vi "testExample_ADC.vi"(8 "error in (no error)":errorcluster, 11 "TestCase in":refnum<class "MyTestCase_shido.lvclass">) -> (0 "error out":errorcluster, 3 "TestCase out":refnum<class "MyTestCase_shido.lvclass">)   [LabVIEW 2020, in "MyTestCase_shido.lvclass"]
doc: "Testea el ejemplo de leer adc de un dispositivo simulado en donde la respuesta esta previamente configurada."
uses:
  MyTestCase_shido.lvclass
  Implementacion/Simulated/Simulated.lvclass
  <vilib>/addons/_JKI Toolkits/VI Tester/TestCase.llb/TestCase.lvclass
  C:/Program Files/National Instruments/LabVIEW 2020/vi.lib/addons/_JKI Toolkits/VI Tester/TestCase.llb/TestCase.lvclass
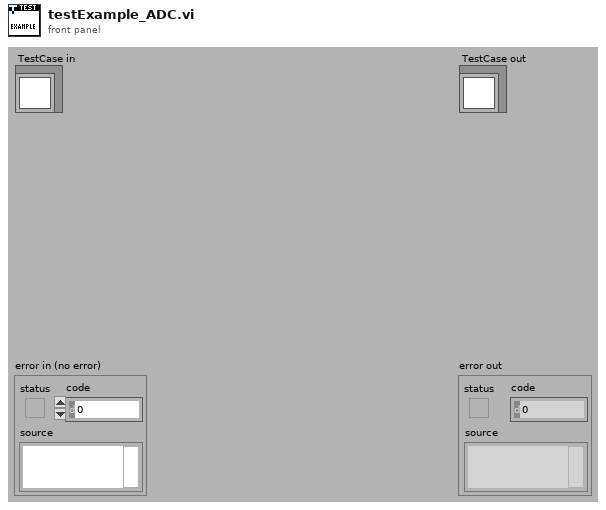
[diagram p1: front panel]
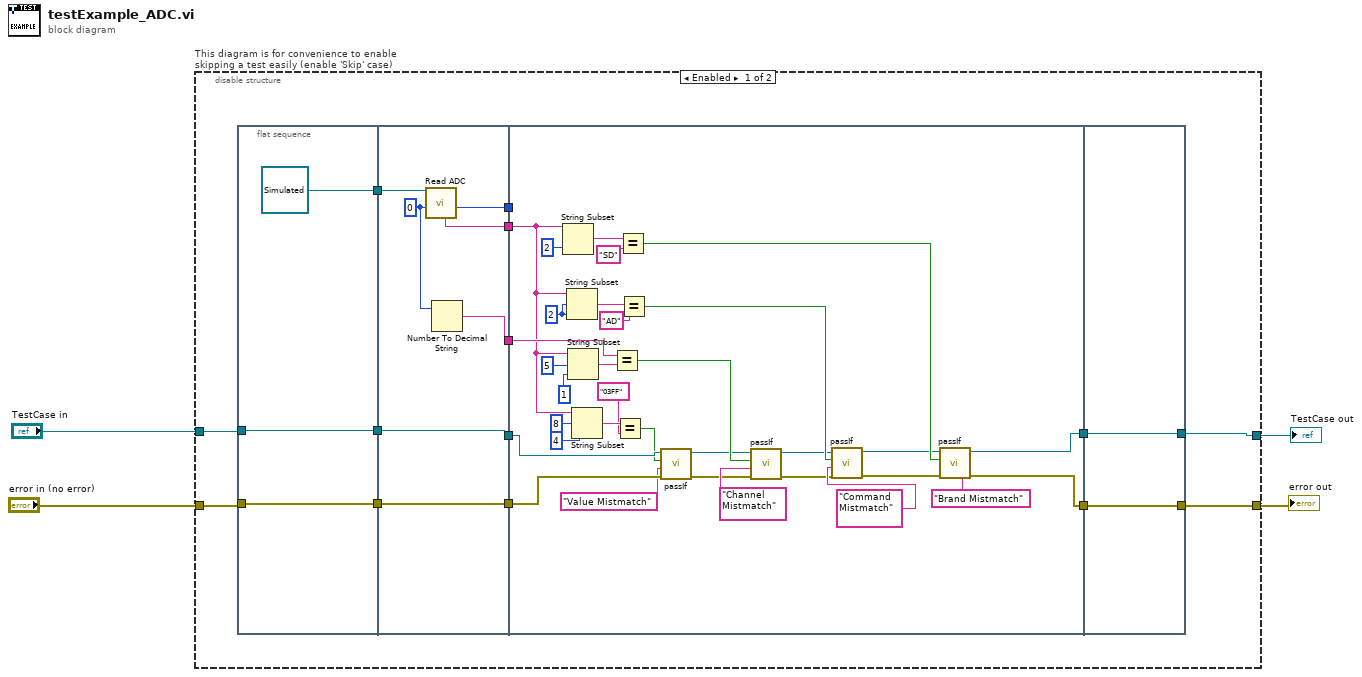
[diagram p0: block diagram]
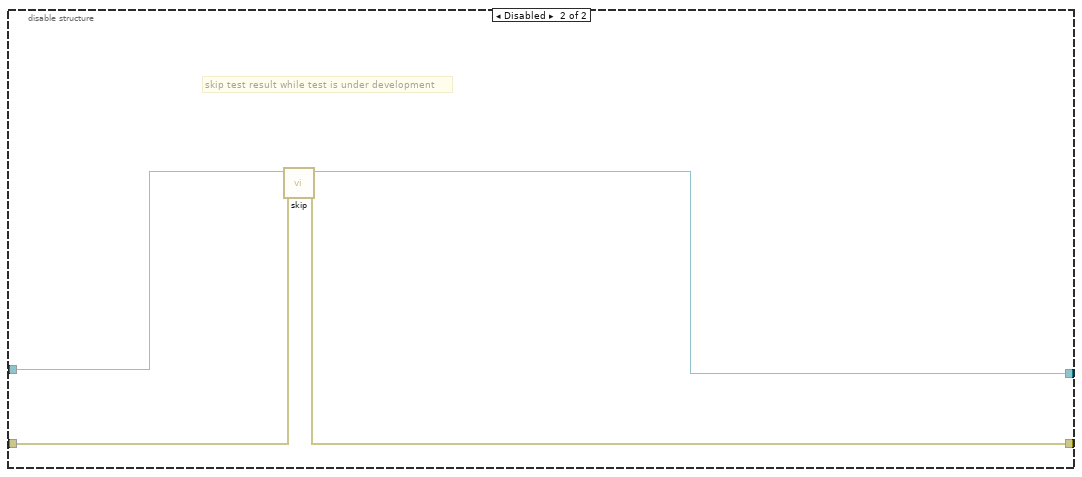
[diagram p2: hidden frame]
diagram:
  n1 = disable-structure "This diagram is for convenience to enable skipping a test easily (enable 'Skip' case)" shown="Enabled" {
    disable-tunnel: "TestCase in" -> [w15 w67]
    disable-tunnel: [w9 w65] -> w1
    disable-tunnel: [w7 w66] -> w3
    disable-tunnel: "error in (no error)" -> [w10 w64]
    frame Enabled {
      n2 = flat-sequence {
        tunnel: [refnum<class "Simulated.lvclass"> refnum ("Simulated.lvclass")] -> w18
        tunnel: w15 -> [w20]
        tunnel: [w20] -> w14
        tunnel: w10 -> [w19]
        tunnel: [w19] -> w12
        tunnel: w18 -> [w28]
        tunnel: [w27] -> w17
        tunnel: [w26] -> w16
        tunnel: w14 -> [w25]
        tunnel: [w25] -> w13
        tunnel: w12 -> [w24]
        tunnel: [w24] -> w11
        tunnel: [w22] -> w5
        tunnel: w17 -> [w38]
        tunnel: w16 -> [_]
        tunnel: w13 -> [w32]
        tunnel: w11 -> [w58]
        tunnel: [w56] -> w8
        tunnel: [w55] -> w6
        tunnel: w5 -> [w43]
        tunnel: [w63] -> w9
        tunnel: w8 -> [w63]
        tunnel: [w62] -> w7
        tunnel: w6 -> [w62]
        frame #0 {
        }
        frame #1 {
          w23 = u8 0 ("Canal")
          n3 = call-dynamic "Read ADC.vi"("Canal"=w23, "Simulated in"=w28) -> ("Response"=w26:i32, "String"=w27:string)  [unwired: 5 in, 3 out]
          n4 = Number To Decimal String(number=w23) -> (decimal integer string=w22:string)  [unwired: 1 in]
        }
        frame #2 {
          w54 = 2 ("length (rest)")
          n5 = String Subset(string=w38, length (rest)=2 ("length (rest)")) -> (substring=w60:string)  [unwired: 1 in]
          n6 = String Subset(string=w38, offset (0)=w54, length (rest)=w54) -> (substring=w47:string)
          n7 = String Subset(string=w38, offset (0)=5, length (rest)=1 ("length (rest)")) -> (substring=w44:string)
          n8 = String Subset(string=w38, offset (0)=8, length (rest)=4 ("length (rest)")) -> (substring=w35:string)
          n9 = Equal?(x=w43, y=w44) -> (x = y?=w40:bool)
          n10 = Equal?(x=w35, y="03FF") -> (x = y?=w30:bool)
          n11 = Equal?(x=w60, y="SD") -> (x = y?=w57:bool)
          n12 = Equal?(x=w47, y="AD") -> (x = y?=w50:bool)
          n13 = call-dynamic "passIf.vi"("error in (no error)"=w58, "message (\"\")"="Value Mistmatch" ("message (\"\")"), "pass"=w30, "TestCase in"=w32) -> ("error out"=w33:errorcluster, "TestCase out"=w31:refnum<class "MyTestCase_shido.lvclass">)  [unwired: 6 in]
          n14 = call-dynamic "passIf.vi"("error in (no error)"=w33, "message (\"\")"="Channel Mistmatch" ("message (\"\")"), "pass"=w40, "TestCase in"=w31) -> ("error out"=w42:errorcluster, "TestCase out"=w41:refnum<class "MyTestCase_shido.lvclass">)  [unwired: 6 in]
          n15 = call-dynamic "passIf.vi"("error in (no error)"=w42, "message (\"\")"="Command Mistmatch" ("message (\"\")"), "pass"=w50, "TestCase in"=w41) -> ("error out"=w52:errorcluster, "TestCase out"=w51:refnum<class "MyTestCase_shido.lvclass">)  [unwired: 6 in]
          n16 = call-dynamic "passIf.vi"("error in (no error)"=w52, "message (\"\")"="Brand Mistmatch" ("message (\"\")"), "pass"=w57, "TestCase in"=w51) -> ("error out"=w55:errorcluster, "TestCase out"=w56:refnum<class "MyTestCase_shido.lvclass">)  [unwired: 6 in]
        }
        frame #3 {
        }
      }
    }
    frame Disabled {
      # "skip test result while test is under development"
      n17 = call <vilib>:"skip.vi"("error in (no error)"=w64, "TestCase in"=w67) -> ("error out"=w66:errorcluster, "TestCase out"=w65:refnum<class "MyTestCase_shido.lvclass">)  [unwired: 8 in]
    }
  }
  "error out" <- w3
  "TestCase out" <- w1
